vi "Dashboard Main.vi"() -> ()   [LabVIEW 2014]
uses:
  <vilib>/event_ctls.llb/eventvkey.ctl
  <vilib>/Rock Robotics/WPI/Dashboard/WPI_DashboardLogging Global.vi
  <vilib>/Rock Robotics/Network Tables/SD Read Numeric Array.vi
  <vilib>/Rock Robotics/Network Tables/SD Write Numeric Array.vi
  <vilib>/Rock Robotics/Network Tables/SD Write String Array.vi
  <vilib>/Rock Robotics/Network Tables/SD Read String Array.vi
  <vilib>/Rock Robotics/Network Tables/SD Write Boolean.vi
  <vilib>/Utility/config.llb/Write Key (String).vi
  <vilib>/Utility/config.llb/Write Key (I32).vi
  <vilib>/Utility/config.llb/NI_LVConfig.lvlib
panel:
  in  "TCP":refnum<k5>
  out "Camera IP":string
  out "Image Message":string="Timeout in Camera Communications"
  in  "Dashboard Tab":T1(tab)
  out "LR":dbl(slide) scale=-1.0..1.0
  out "RR":dbl(slide) scale=-1.0..1.0
  out "RF":dbl(slide) scale=-1.0..1.0
  out "LF":dbl(slide) scale=-1.0..1.0
  in  "Camera Settings":T2={"Frame Rate"=30, "Compression"=30, "Size"=1} {"Frame Rate" scale=1.0..30.0; "Size" items=["640x480", "320x240", "160x120"]}
  out "Mode":T3(ring)=enum."Auto Disabled"
  in  "DB Camera Config":bool
  out "fps":dbl format="%#.1g"
  out "Mbps":dbl format="%#.1g"
  out "Mbps 2":bool
  out "HID":T4(array[cluster])
  out "Time until start/end":sgl
  in  "DB/String 9":string
  in  "DB/String 8":string
  in  "DB/String 7":string
  in  "DB/String 6":string
  in  "DB/String 5":string
  in  "DB/String 4":string
  in  "DB/String 3":string
  in  "DB/String 2":string
  in  "DB/String 1":string
  in  "DB/String 0":string
  in  "DB/Slider 0":dbl(slide) scale=0.0..5.0
  in  "DB/Slider 1":dbl(slide) scale=0.0..5.0
  in  "DB/Slider 2":dbl(slide) scale=0.0..5.0
  in  "DB/Slider 3":dbl(slide) scale=0.0..5.0
  out "DB/LED 3":bool
  out "DB/LED 2":bool
  out "DB/LED 1":bool
  out "DB/LED 0":bool
  in  "DB/Button 3":bool
  in  "DB/Button 2":bool
  in  "DB/Button 1":bool
  in  "DB/Button 0":bool caption="New Name"
  in  "Rec Mode":enum32{"Stop", "Record", "Playback"}(radio)
  in  "Vision":u16(ring) items=["Camera Off", "USB Camera SW", "USB Camera HW", "IP Camera"]
  in  "Translate X":T5(ring)
  in  "Translate Y":T5(ring)=enum."Y left"
  in  "Rotate":T5(ring)=enum."X right"
  in  "Gyro Reset":T6(ring)
  in  "Toggle Field Centric":T6(ring)=enum."Trigger Right"
  in  "Low elevator":T7(ring)=enum."Left bumper"
  in  "Axis for manual Control of \narm":T8(ring)
  in  "High elevator":T7(ring)=enum."Right bumper"
  in  "Claw up":T7(ring)
  in  "Claw Down":T7(ring)=enum."B"
  in  "Axis for manual Control of Claw":T8(ring)
  in  "Rotate Claw":T9(ring)=enum."Right trigger"
  in  "Open/Close claw":T7(ring)=enum."Y"
  in  "Test Slider":dbl(slide) scale=0.0..100.0 scale format="%#_3g"
  in  "On/Off":bool caption="Solenoid"
  in  "Test Name":u16(ring) items=["Select the test to run...", "Example Test", "-------------------------------", "List of tests is built in robot code.", "Replace with your own automated tests."]
  in  "Test Tree":string(tree)
  in  "Motor":cluster{"Value":dbl, "Enable":bool} {"Value" scale=-1.0..1.0 scale format="%#_3g"}
  out "Progress":T10 {"Test Progress" scale=0.0..100.0}
  in  "Rev/Fwd":cluster{"Forward":bool, "Reverse":bool}
  in  "Test Ring":u16(ring) items=["Monochrome", "Color"]
  in  "Listbox":i32(listbox)
  in  "?":bool
  in  "Variables":string[](array[string])
  out "Camera Image":T11(plugin-control)
  out "Boolean":bool
  # "Battery"
  # "Primary Driver"
  # "Axis controls"
  # "Button Controls"
  # "Secondary Driver"
  # "Axis controls"
  # "Button Controls"
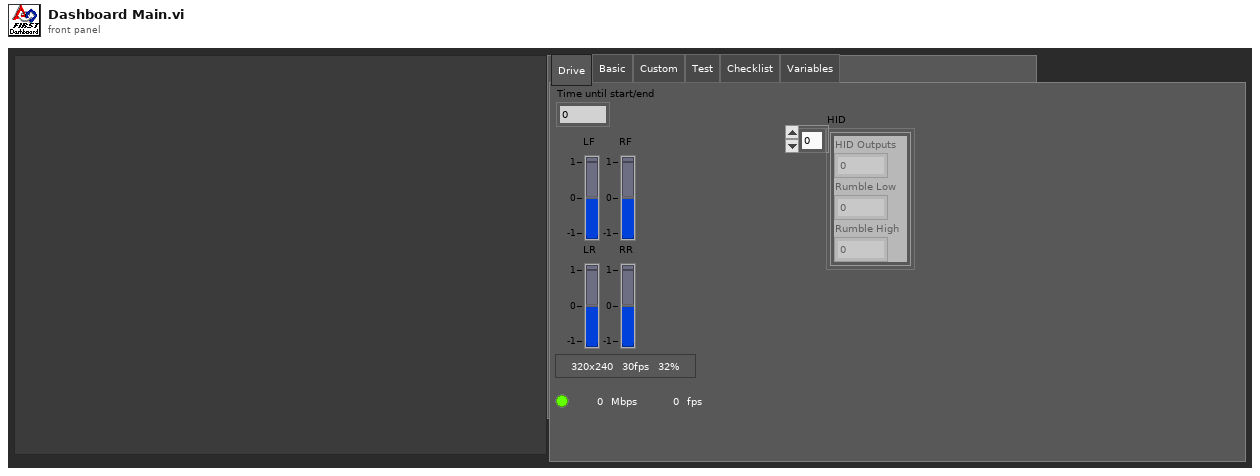
[diagram p1: front panel]
types:
  T1 = enum32{"Drive", "Basic", "Custom", "Test", "Checklist", "Variables"}
  T2 = cluster{"Frame Rate":i32, "Compression":i32, "Size":u16}
  T3 = enum8{"Tele-Op Disabled", "Tele-Op Enabled", "Auto Disabled", "Auto Enabled", "Test Disabled", "Test Enabled", "Disconnected", "No Code", "E-Stop"}
  T4 = cluster{"HID Outputs":u32, "Rumble Low":u16, "Rumble High":u16}[]
  T5 = enum16{"X left ", "Y left", "Z left", "X right", "Y right", "Z right"}
  T6 = enum16{"Trigger Left", "2 Left", "3 Left", "4 Left", "5 Left", "6 Left", "7 Left", "8 Left", "9 Left", "10 Left", "11 Left", "Trigger Right", "2 Right", "3 Right", "4 Right", "5 Right", "6 Right", "7 Right", "8 Right", "9 Right", "10 Right", "11 Right"}
  T7 = enum16{"A", "B", "X", "Y", "Left bumper", "Right bumper", "Back", "Start", "Left Joystick down", "Right Joystick down"}
  T8 = enum16{"Left X", "Left Y", "Left trigger", "R trigger", "R X", "R Y"}
  T9 = enum16{"Left X", "Left Y", "Left trigger", "Right trigger", "Right X", "Right Y"}
  T10 = cluster{"Test Progress":u8, "Test Progress Text":string}
  T11 = typedef "IMAQ Image.ctl" = refnum<image>
  T12 = typedef "Image Type" = u32
  T13 = cluster{"Error Strings":string, "Disable Counts":cluster{u16, u16}, "Rail Faults":cluster{u16, u16, u16}, "Robot IP":string, "DB Mode":u8, "Event Info":cluster{"Name":string, "Type":u8, "Number":u16, "Replay":u8}, "Camera Addr":string}
  T14 = cluster{"Storage":cluster{"Disk Free":u64, "RAM Block":u32, "RAM free":u32}, "CPU Utilization":cluster{"CPU % ISR":sgl, "CPU % Time Crit":sgl, "CPU % Timed Str":sgl, "CPU % High":sgl, "CPU % Above":sgl, "CPU % Normal":sgl, "CPU % Low":sgl}, "CAN":cluster{"% Bus Utilization":sgl, "Bus Off Cnt":u32, "TX_FIFO Full Cnt":u32, "Receive Error Cnt":u8, "Transmit Error Cnt":u8}, "HID":cluster{"HID Outputs":u32, "Rumble Low":u16, "Rumble High":u16}[]}
  T15 = cluster{"Status bits":cluster{"Test Mode":bool, "Autonomous":bool, "Enabled":bool, "Code Start":bool, "Brownout":bool, "Reserved 2":bool, "Reserved 3":bool, "E-Stop":bool}, "Code Trace":cluster{"Disabled":bool, "TeleOp":bool, "Auto":bool, "Test":bool}, "Controller Type":enum16{"unknown", "cRIO", "roboRio"}, "Code?":enum16{"unknown", "noCode", "code"}, "Battery V":dbl}
  T16 = cluster{"Control Bits":cluster{"TestMode":bool, "Autonomous":bool, "Enabled":bool, "FMS Present":bool, bool, bool, bool, "E-Stop":bool}, "Team Station ":u8, "Countdown":sgl, "Joystick Values":cluster{"Axes":dbl[], "Buttons":bool[], "POVs":i16[]}[]}
  T17 = enum16{"X left ", "Y left", "Z left", "X right", "Y right", "Z right"}[]
  T18 = enum16{"A", "B", "X", "Y", "Left bumper", "Right bumper", "Back", "Start", "Left Joystick down", "Right Joystick down"}[]
  T19 = enum16{"Trigger Left", "2 Left", "3 Left", "4 Left", "5 Left", "6 Left", "7 Left", "8 Left", "9 Left", "10 Left", "11 Left", "Trigger Right", "2 Right", "3 Right", "4 Right", "5 Right", "6 Right", "7 Right", "8 Right", "9 Right", "10 Right", "11 Right"}[]
  T20 = typedef "NI_LVConfig.lvlib/Config Data RefNum.ctl" = refnum<k1>
  T21 = cluster{"Operation":enum16{"Update", "Clear"}, "Color Box":u32}[]
  T22 = typedef "eventvkey.ctl" = enum16{"ASCII", "Enter", "Return", "Shift", "Ctrl", "Alt", "Cmd", "Opt", "Caps", "NumLock", "Clear", "Break", "Up", "Down", "Left", "Right", "Insert", "Delete", "Home", "End", "PageUp", "PageDown", "Escape", "Help", "Pause", "ScrollLock", "F1", "F2", "F3", "F4", "F5", "F6", "F7", "F8", "F9", "F10", "F11", "F12", "F13", "F14", "F15", "F16", "F17", "F18", "F19", "F20", "F21", "F22", "F23", "F24", "Play", "VolumeUp", "VolumeDown", "Mute", "Two Byte Char"}
  T23 = cluster{"Image Size":bool, "Image Type":bool, "Pixel Value":bool, "ROI Information":bool, "Zoom Factor":bool}
  T24 = enum8{"Enabled", "Disabled", "Disabled and Grayed Out"}
  T25 = cluster{"Operation":enum16{"Update", "Clear"}, "Color Box":u32}
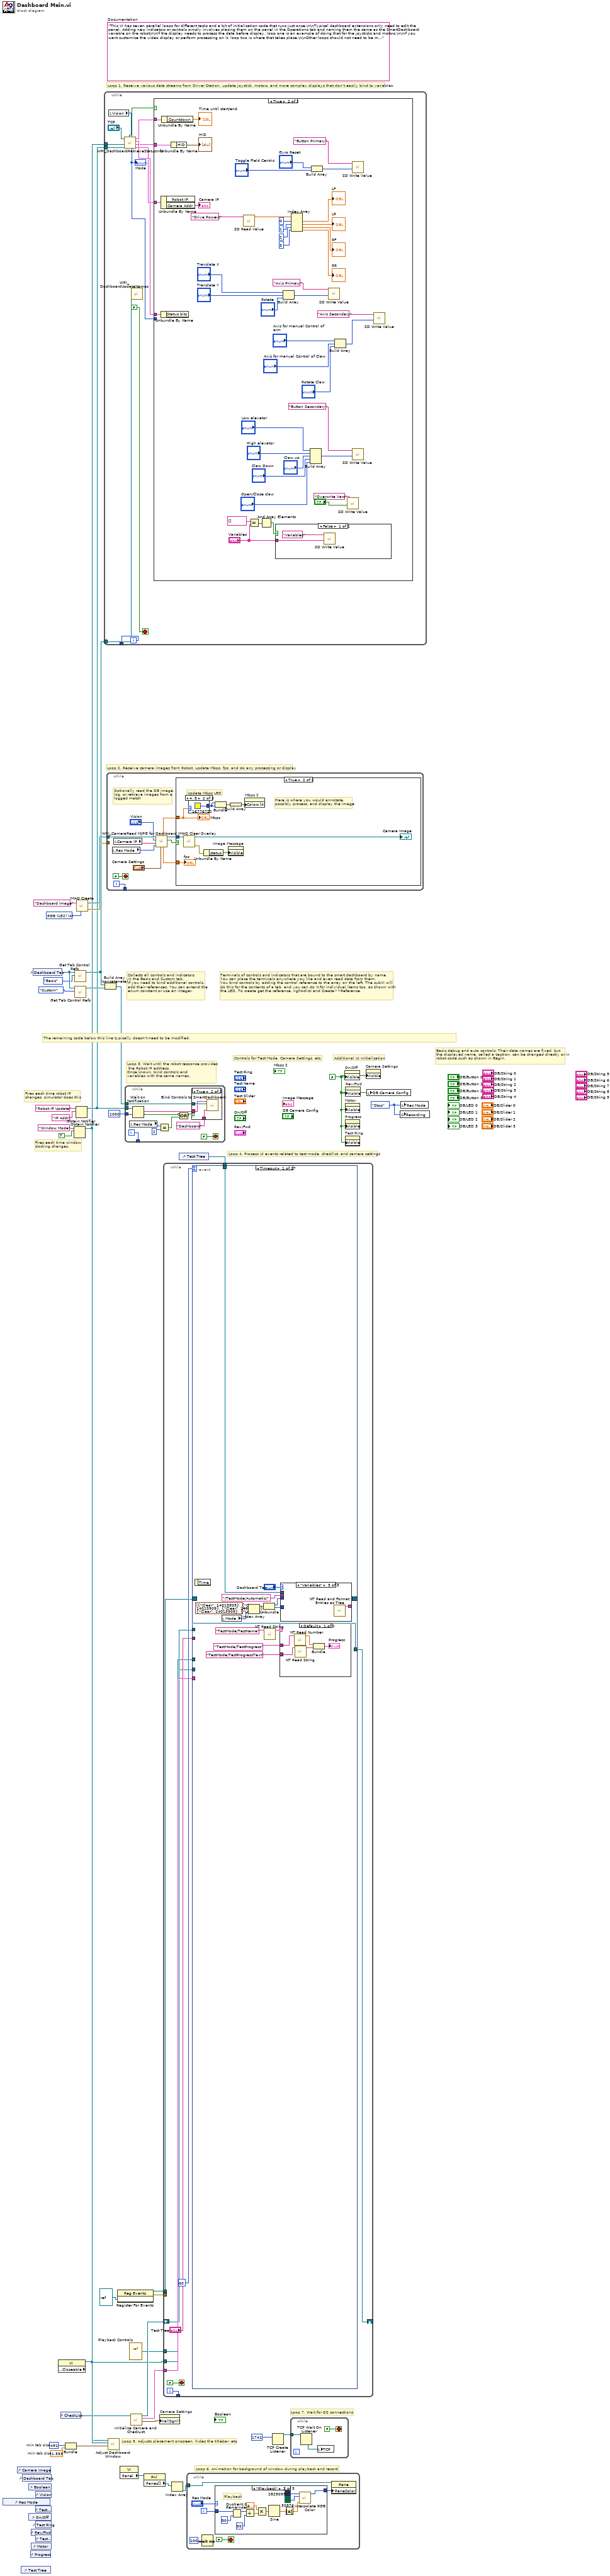
[diagram p0: block diagram]
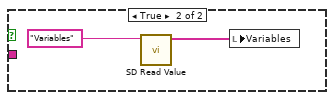
[diagram p3: hidden frame]
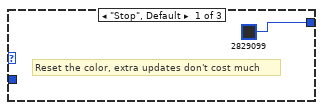
[diagram p4: hidden frame]
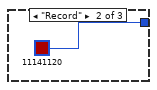
[diagram p5: hidden frame]
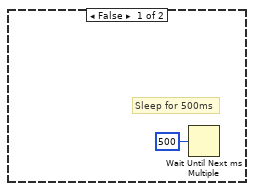
[diagram p7: hidden frame]
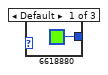
[diagram p8: hidden frame]
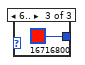
[diagram p9: hidden frame]
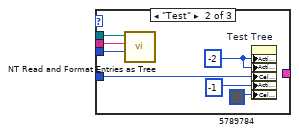
[diagram p11: hidden frame]
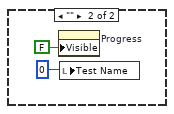
[diagram p12: hidden frame]
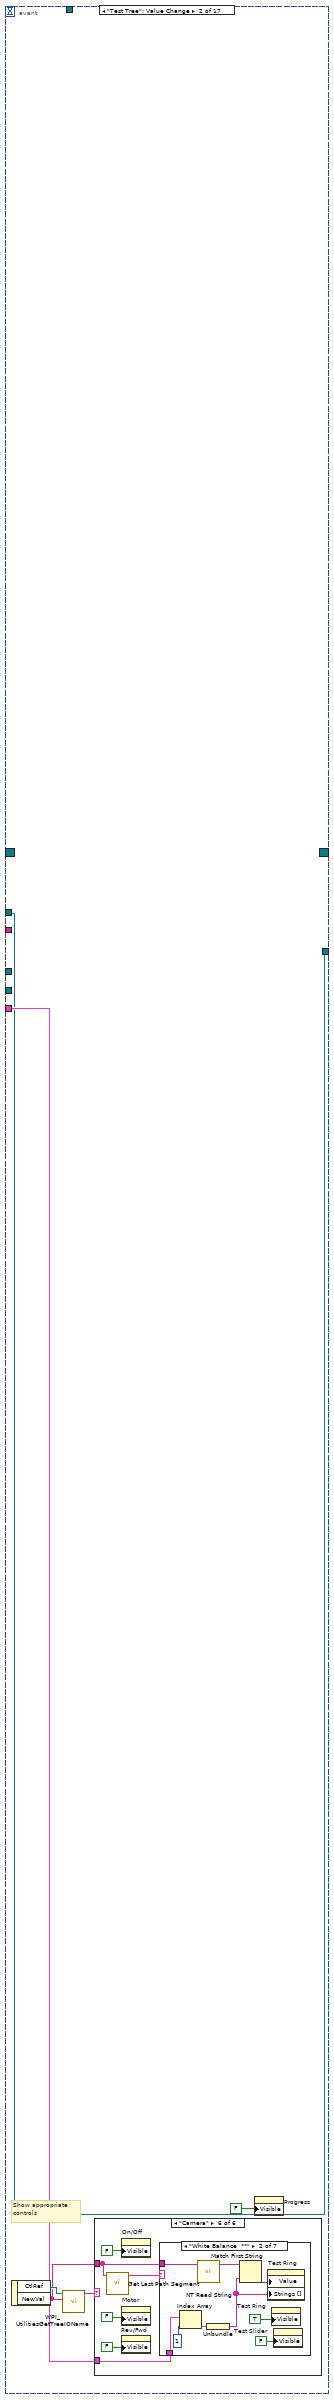
[diagram p13: hidden frame]
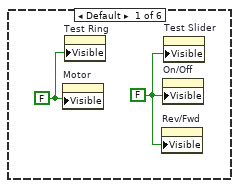
[diagram p14: hidden frame]
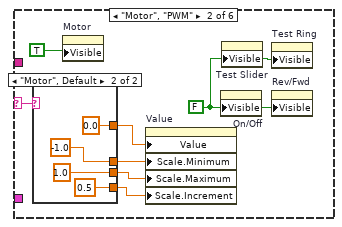
[diagram p15: hidden frame]
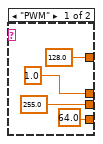
[diagram p16: hidden frame]
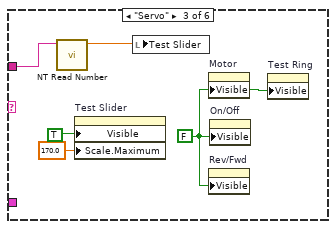
[diagram p17: hidden frame]
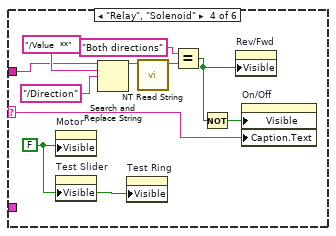
[diagram p18: hidden frame]
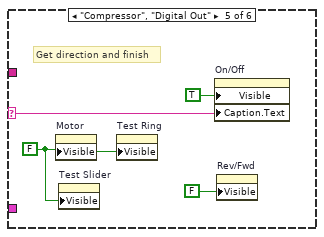
[diagram p19: hidden frame]
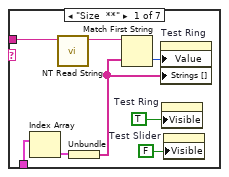
[diagram p20: hidden frame]
diagram:
  w12 = 491  # min tab size
  w11 = 1.333  # min tab size
  w17 = enum32{"Stop", "Record", "Playback"}."Stop" ("Rec Mode")
  w6 = FALSE ("Visible")
  (unwired) "This VI has seven parallel loops for different tasks and a bit of initialization code that runs just once.\n\nTypical dashboard extensions only need to edit the panel. Adding new indicators or controls simply involves placing them on the panel in the Operations tab and naming them the same as the SmartDashboard variable on the robot\n\nIf the display needs to process the data before display, loop one is an example of doing that for the joysticks and motors.\n\nIf you want customize the video display or perform processing on it, loop two is where that takes place.\n\nOther loops should not need to be modified. They are pretty standard, and document the task they perform."  # Documentation
  w37 = T12 4 items=["Grayscale (U8)", "Grayscale (I16)", "Grayscale (SGL)", "Complex (CSG)", "RGB (U32)", "HSL (U32)", "RGB (U64)"] ("Image Type")
  # "Loop 7. Wait for DS connections"
  # "Basic debug and auto controls: Their data names are fixed, but\nthe displayed name, called a caption, can be changed directly or in\nrobot code such as shown in Begin."
  # "Controls for Test Mode, Camera Settings, etc."
  # "Additional UI Initialization"
  # "Loop 6. Animation for background of window during playback and record"
  # "Fires each time robot IP\nchanges, simulator does this"
  # "Fires each time window\ndocking changes."
  # "Collects all controls and indicators\nin the Basic and Custom tab.\nIf you need to bind additional controls,\nadd their references. You can extend the\nenum constant or use an integer."
  # "The remaining code below this line typically doesn't need to be modified."
  # "Loop 4. Process UI events related to test mode, checklist, and camera settings"
  # "Terminals of controls and indicators that are bound to the smart dashboard by name.\nYou can place the terminals anywhere you like and even read data from them.\nYou bind controls by adding the control reference to the array on the left. The subVI will\ndo this for the contents of a tab, and you can do it for individual items too, as shown with\nthe LED. To create get the reference, right-click and Create>>Reference."
  # "Loop 3. Wait until the robot response provides\n the Robot IP address.\nOnce known, bind controls and\nvariables with the same names."
  # "Loop 5. Adjusts placement onscreen, hides the titlebar, etc."
  # "Loop 1. Receive various data streams from Driver Station, update joystick, motors, and more complex displays that don't easily bind to variables."
  # "Loop 2. Receive camera images from Robot, update Mbps, fps, and do any processing or display"
  n1 = control-ref of="Rec Mode"() -> ()  [unwired: 1 out]
  n2 = control-ref of="Camera Image"() -> ()  [unwired: 1 out]
  n3 = control-ref of="Test Tree"() -> ()  [unwired: 1 out]
  n4 = control-ref of="Dashboard Tab"() -> ()  [unwired: 1 out]
  n5 = control-ref of="Boolean"() -> ()  [unwired: 1 out]
  n6 = control-ref of="On/Off"() -> ()  [unwired: 1 out]
  n7 = control-ref of="Progress"() -> ()  [unwired: 1 out]
  n8 = control-ref of="Rev/Fwd"() -> ()  [unwired: 1 out]
  n9 = control-ref of="Motor"() -> ()  [unwired: 1 out]
  n10 = control-ref of="Dashboard Tab"() -> (w15:refnum<vi>)
  n11 = control-ref of="Test Slider"() -> ()  [unwired: 1 out]
  n12 = control-ref of="Vision"() -> ()  [unwired: 1 out]
  n13 = control-ref of="Test Ring"() -> ()  [unwired: 1 out]
  n14 = control-ref of="Test Name"() -> ()  [unwired: 1 out]
  n15 = property class="VI" props=["Front Panel.Closeable"]() -> (reference out=w16:refnum<vi>)  [unwired: 2 in, 2 out]
  n16 = control-ref of="CheckList"() -> (w7:refnum<vi>)
  n17 = Bundle("min tab size"=w12, "min tab size"=w11) -> (w10:cluster{"min tab size":i32, "min tab size":dbl})  [unwired: 1 in]
  n18 = Obtain Notifier(name (unnamed)="Window Mode", notification data type=TRUE) -> (notifier out=w3:refnum<notifier>)  [unwired: 2 in, 2 out]
  n19 = call <vilib>:"Get Tab Control Refs.vi"("Page Index"=T1."Basic" ("Dashboard Tab"), "TabControl in"=w15) -> ("ControlsOnPage"=w4:refnum<vi>[])  [unwired: 9 in]
  n20 = call <vilib>:"Get Tab Control Refs.vi"("Page Index"=T1."Custom" ("Dashboard Tab"), "TabControl in"=w15) -> ("ControlsOnPage"=w14:refnum<vi>[])  [unwired: 9 in]
  n21 = Obtain Notifier(name (unnamed)="Robot IP Update", notification data type="IP Addr" ("name (unnamed)")) -> (notifier out=w5:refnum<notifier>)  [unwired: 2 in, 2 out]
  n22 = call "IMAQ Create"("Image Name"="Dashboard Image", "Image Type"=w37) -> ("New Image"=w35:T11, "error out"=w34:errorcluster)  [unwired: 2 in, 1 out]
  n23 = while {
    tunnel: [w49] -> _
    tunnel: w5 -> [w43]
    tunnel: w4 -> [w42]
    tunnel: w3 -> [w38]
    i -> [w49]
    stop <- FALSE stop-if-true
    n24 = local read "Vision"() -> (w40:u16)
    n25 = call <vilib>:"WPI_DashboardRetrieveStatusInfo.vi"("Vision"=w40, "Binding Refnum"=w43, "Window Mode Notifier"=w38, "TCP Cnx"="TCP") -> ("Power and Errors"=w44:T13, "Robot Metrics"=w47:T14, "Status Info"=w48:T15, "Control Info"=w45:T16, "Robot Mode"=w41:T3, "Process?"=w46:bool)  [unwired: 2 in]
    "Mode" <- w41
    n26 = call <vilib>:"WPI_DashboardUpdateNames.vi"("Controls on Tab"=w42) -> ()  [unwired: 11 in]
    n27 = case shown="True" w46 {
      tunnel: w48 -> [_ w94]
      tunnel: w47 -> [_ w93]
      tunnel: w45 -> [_ w92]
      tunnel: w44 -> [_ w91]
      tunnel: w41 -> [_ _]
      frame False {
      }
      frame True {
        n28 = Unbundle By Name(w91) -> ("Camera Addr"=→"Camera IP":string)  [unwired: 1 out]
        n29 = Unbundle By Name(w94) -> ()  [unwired: 1 out]
        n30 = Unbundle By Name(w92) -> ("Countdown"=→"Time until start/end":sgl)
        n31 = Unbundle By Name(w93) -> ("HID"=→"HID":T4)
        n32 = call-poly <vilib>:"SD Read Value.vi"("Name"="Drive Powers") -> ("Numeric Array"=w86:dbl[])  [unwired: 8 in, 2 out]
        n33 = Equal?(x=string[] [], y="Variables") -> (x = y?=w55:bool[])
        n34 = And Array Elements(Boolean array=w55) -> (logical AND=w54:bool)
        n35 = case shown="False" w54 {
          tunnel: "Variables" -> [w95 _]
          frame False {
            n36 = call-poly <vilib>:"SD Write Value.vi"("String Array"=w95, "Name"="Variables") -> ()  [unwired: 8 in, 2 out]
          }
          frame True {
            n37 = call-poly <vilib>:"SD Read Value.vi"("Name"="Variables") -> ("String Array"=w97:string[])  [unwired: 9 in, 1 out]
            n38 = local write "Variables"(w97) -> ()
          }
        }
        n39 = Build Array("Translate X", "Translate Y", "Rotate") -> (w75:T17)
        n40 = Index Array(array=w86, index #1=0 ("index"), index #2=1 ("index"), index #3=2 ("index"), index #4=3 ("index")) -> (element #1=→"LF":dbl, element #2=→"LR":dbl, element #3=→"RF":dbl, element #4=→"RR":dbl)
        n41 = Build Array("Low elevator", "High elevator", "Claw up", "Claw Down", "Open/Close claw") -> (w66:T18)
        n42 = Build Array("Gyro Reset", "Toggle Field Centric") -> (w71:T19)
        n43 = call-poly <vilib>:"SD Write Value.vi"("Numeric Array"=w75, "Name"="Axis Primary") -> ()  [unwired: 8 in, 2 out]
        n44 = Build Array("Axis for manual Control of \narm", "Axis for manual Control of Claw", "Rotate Claw") -> (w68:u16[])
        n45 = call-poly <vilib>:"SD Write Value.vi"("Boolean"="?", "Name"="Overwrite Vars") -> ()  [unwired: 8 in, 2 out]
        n46 = call-poly <vilib>:"SD Write Value.vi"("Numeric Array"=w71, "Name"="Button Primary") -> ()  [unwired: 8 in, 2 out]
        n47 = call-poly <vilib>:"SD Write Value.vi"("Numeric Array"=w66, "Name"="Button Secondary") -> ()  [unwired: 8 in, 2 out]
        n48 = call-poly <vilib>:"SD Write Value.vi"("Numeric Array"=w68, "Name"="Axis Secondary") -> ()  [unwired: 8 in, 2 out]
      }
    }
  }
  n49 = Build Array (concatenate)(w4, w14) -> (w13:refnum<vi>[])
  n50 = while {
    tunnel: w35 -> [w107]
    tunnel: w34 -> [_]
    tunnel: [w108] -> _
    i -> [w108]
    stop <- FALSE stop-if-true
    # "Optionally read the DB image,\nlog, or retrieve images from a\nlogged match"
    n51 = local read "Rec Mode"() -> (w101:enum32{"Stop", "Record", "Playback"})
    n52 = local read "Camera IP"() -> (w99:string)
    n53 = call <vilib>:"WPI_CameraRead MJPG for Dashboard.vi"("Camera Settings"="Camera Settings", "Rec Mode"=w101, "Camera IP"=w99, "Camera Mode"="Vision", "Refnum in"=w107) -> ("Active"=w105:bool, "Refnum out"=w106:T11, "FPS"=w104:dbl, "Bandwidth (Mbps)"=w103:dbl)  [unwired: 3 in]
    n54 = case shown="True" w105 {
      tunnel: w106 -> [_ w114]
      tunnel: w103 -> [_ w113]
      tunnel: w104 -> [_ w111]
      frame False {
        # "Sleep for 500ms"
        n55 = Wait Until Next ms Multiple(millisecond multiple=u32 500) -> ()  [unwired: 1 out]
      }
      frame True {
        # "Here is where you would annotate,\npossibly process, and display the image"
        # "Update Mbps LED"
        n56 = call "IMAQ Clear Overlay"("Image"=w114) -> ("error out"=w118:errorcluster, "Image Out"=→"Camera Image":T11)  [unwired: 2 in, 7 out]
        n57 = case shown="4, 5" w113 {
          tunnel: [u32 6618880 ("Color Box") u32 16776722 ("Color Box") u32 16716800 ("Color Box")] -> w115
          frame Default {
          }
          frame 4, 5 {
          }
          frame 6.. {
          }
        }
        n58 = Unbundle By Name(w118) -> ("status"=w119:bool)
        n59 = Bundle("Color Box"=w115, "Color Box"=w115) -> (w117:cluster{"Color Box":u32, "Color Box":u32})  [unwired: 1 out]
        n60 = property on="Image Message" class="Str"("Visible"=w119) -> ()  [unwired: 2 in, 2 out]
        n61 = Build Array(w117) -> (w116:cluster{"Color Box":u32, "Color Box":u32}[])
        n62 = property on="Mbps 2" class="Bool (strict)"("Colors [4]"=w116) -> ()  [unwired: 2 in, 2 out]
        "Mbps" <- w113
        "fps" <- w111
      }
    }
  }
  n63 = call "Adjust Dashboard Window.vi"("Size Constraints"=w10, "VI"=w16, "Notifier in"=w3) -> ()  [unwired: 9 in]
  n64 = register-events(refnum<vi> refnum) -> (reference out=w21:refnum<event-registration>, error out=w20:errorcluster)  [unwired: 2 in]
  n65 = property class="VI"() -> ("Panel"=w24:refnum<vi>)  [unwired: 2 in, 2 out]
  n66 = while {
    tunnel: w13 -> [w134]
    tunnel: w5 -> [w132]
    tunnel: [w130] -> _
    tunnel: u32 1000 ("milliseconds to wait") -> [w129]
    i -> [w130]
    stop <- FALSE stop-if-true
    n67 = local read "Rec Mode"() -> (w125:enum32{"Stop", "Record", "Playback"})
    n68 = Wait on Notification(notifier=w132, timeout in ms (-1)=w129) -> (notification=w131:string, timed out?=w127:bool)  [unwired: 2 in, 2 out]
    n69 = Equal?(x=w125, y=u16 2 ("Rec Mode")) -> (x = y?=w126:bool)
    n70 = Compound Arithmetic op=OR(invert w127, w126) -> (w128:bool)
    n71 = case shown="True" w128 {
      tunnel: w134 -> [_ w137]
      tunnel: w131 -> [_ w136]
      tunnel: "Dashboard" -> [_ w135]
      frame False {
      }
      frame True {
        n72 = call <vilib>:"Bind Controls to SmartDashboard.vi"("Client Name"=w135, "Bound Control Refs"=w137, "Server IP Address"=w136) -> ()  [unwired: 9 in]
      }
    }
  }
  n73 = vi-ref "Playback Controls.vi"() -> (w22:refnum<vi>)
  n74 = call "Initialize Camera and CheckList.vi"("ListBox in"=w7) -> ("Cluster"=w28:cluster{"value":i32, "value":i32, "index":i32}, "Array"=w29:cluster{string[]}[], "File Refnum"=w27:T20)  [unwired: 8 in]
  n75 = property class="Pnl"(reference=w24) -> ("Panes[]"=w25:refnum<vi>[])  [unwired: 1 in, 2 out]
  n76 = property on="Camera Settings" class="Clust (strict)"("Val(Sgnl)"=w28) -> ()  [unwired: 2 in, 2 out]
  n77 = Index Array(array=w25) -> (element=w23:refnum<vi>)  [unwired: 1 in]
  n78 = control-ref of="Test Tree"() -> (w26:refnum<vi>)
  n79 = while {
    tunnel: w29 -> [w145]
    shift-right: [w144] -> _
    shift-left: w27 -> [w143]
    tunnel: [w142] -> _
    tunnel: w26 -> [w141]
    tunnel: w22 -> [w140]
    tunnel: w21 -> [w139]
    tunnel: w20 -> [_]
    tunnel: w16 -> [w138]
    i -> [w142]
    stop <- FALSE stop-if-true
    n80 = event shown="[0] Timeout" {
      selector: w139 -> [_ _ _ _ _ _ _ _ _ _ _ _ _ _ _ _ _]
      dyn-events: [_ _ _ _ _ _ _ _ _ _ _ _ _ w382 _ _ _] -> _
      timeout: u32 60 ("milliseconds to wait") -> [_ _ _ _ _ _ _ _ _ _ _ _ _ _ _ _ _]
      tunnel: w141 -> [w157 _ _ _ _ _ _ _ _ _ _ _ _ _ _ _ _]
      tunnel: "Test Tree" -> [_ _ _ _ _ _ _ _ w351 w359 w361 w365 w373 _ _ _ _]
      tunnel: w145 -> [_ w178 _ _ _ _ w315 w345 _ _ _ _ _ _ _ _ _]
      tunnel: [w153 w177 w276 w281 w289 w301 w314 w338 w350 w357 w360 w364 w372 w384 w398 w399 w409] -> w144
      tunnel: w143 -> [w153 w177 w276 w281 w289 w301 w313 w338 w350 w357 w360 w364 w372 w384 w398 w399 w409]
      tunnel: w140 -> [_ _ _ _ _ _ _ _ _ _ _ _ _ w385 _ w402 _]
      tunnel: w138 -> [_ _ _ _ _ _ _ _ _ _ _ _ _ w380 _ _ _]
      event Timeout {
        n81 = event-data() -> ()  [unwired: 1 in, 1 out]
        n82 = local read "Mode"() -> (w156:T3)
        n83 = Index Array(array=T21 [{"Operation"=enum."Clear", "Color Box"=14013909}, {"Operation"=enum."Clear", "Color Box"=14013909}, {"Operation"=enum."Clear", "Color Box"=14013909}, {"Operation"=enum."Clear", "Color Box"=14013909}, {"Operation"=enum."Update", "Color Box"=14013909}, {"Operation"=enum."Update", "Color Box"=16777215}, {"Operation"=enum."Clear", "Color Box"=14013909}, {"Operation"=enum."Clear", "Color Box"=14013909}, {"Operation"=enum."Clear", "Color Box"=14013909}], index=w156) -> (element=w151:T25)
        n84 = Unbundle(w151) -> ("Operation"=w150:enum16{"Update", "Clear"}, "Color Box"=w149:u32)
        n85 = call <vilib>:"NT Read String.vi"("Name"="TestMode/TestName") -> ("String"=w160:string)  [unwired: 9 in, 1 out]
        n86 = case shown="Default" w160 {
          tunnel: "TestMode/TestProgress" ("Name") -> [w171 _]
          tunnel: "TestMode/TestProgressText" ("Name") -> [w170 _]
          frame Default {
            n87 = call <vilib>:"NT Read Number.vi"("Name"=w171) -> ("Numeric"=w172:dbl)  [unwired: 9 in, 1 out]
            n88 = call <vilib>:"NT Read String.vi"("Name"=w170) -> ("String"=w173:string)  [unwired: 9 in, 1 out]
            n89 = Bundle("Numeric"=w172, "String"=w173) -> (→"Progress":cluster{"Numeric":dbl, "String":string})  [unwired: 1 in]
          }
          frame "" {
            n90 = property on="Progress" class="Clust (strict)"("Visible"=FALSE) -> ()  [unwired: 2 in, 2 out]
            n91 = local write "Test Name"(u16 0) -> ()
          }
        }
        n92 = case shown="\"Variables\"" "Dashboard Tab" {
          tunnel: w157 -> [_ w168 _]
          tunnel: "/TestMode/Automatic/" ("Name Pattern") -> [_ w167 _]
          tunnel: w150 -> [_ w166 _]
          tunnel: [_ _ w169] -> _
          tunnel: w149 -> [_ w162 _]
          frame "Custom", Default {
          }
          frame "Test" {
            w165 = -2 ("Active Item:Row Number")
            n93 = call <vilib>:"NT Read and Format Entries as Tree.vi"("Operation"=w166, "Name Pattern"=w167, "Tree Refnum"=w168) -> ()  [unwired: 7 in, 2 out]
            n94 = property on="Test Tree" class="Tree (strict)"("Active Item Row Number"=w165, "ActiveColNum"=w165, "CellBG"=w162, "Active Item Row Number"=-1 ("Active Item:Row Number"), "CellBG"=u32 5789784 ("Color Box")) -> ()  [unwired: 2 in, 2 out]
          }
          frame "Variables" {
            n95 = call <vilib>:"NT Read and Format Entries as Tree.vi"() -> ("Formatted Strings"=w169:cluster{"Name":string, "Value":string}[])  [unwired: 10 in, 1 out]
          }
        }
      }
      event "Test Tree": Value Change {
        # "Show appropriate\ncontrols"
        n96 = event-data() -> ("CtlRef"=w181:refnum<vi>, "NewVal"=w179:string)  [unwired: 1 in]
        n97 = call <vilib>:"WPI_UtilitiesGetTreeIOName.vi"("NewVal"=w179, "TreeControl in"=w181) -> ("I/O Name"=w182:string)  [unwired: 9 in]
        n98 = case shown="\"Camera\"" w182 {
          selector: w182 -> [_ w189 _ w207 w216 _]
          tunnel: w179 -> [_ _ w204 w206 _ w223]
          tunnel: w178 -> [_ _ _ _ _ w222]
          frame Default {
            w184 = FALSE ("Visible")
            w183 = FALSE ("Visible")
            n99 = property on="Motor" class="Clust (strict)"("Visible"=w183) -> ()  [unwired: 2 in, 2 out]
            n100 = property on="Test Ring" class="Ring (strict)"("Visible"=w183) -> ()  [unwired: 2 in, 2 out]
            n101 = property on="Rev/Fwd" class="Clust (strict)"("Visible"=w184) -> ()  [unwired: 2 in, 2 out]
            n102 = property on="On/Off" class="Bool (strict)"("Visible"=w184) -> ()  [unwired: 2 in, 2 out]
            n103 = property on="Test Slider" class="Slide (strict)"("Visible"=w184) -> ()  [unwired: 2 in, 2 out]
          }
          frame "Motor", "PWM" {
            w190 = FALSE ("Visible")
            n104 = case shown="\"Motor\", Default" w189 {
              tunnel: [1.0 ("Value") -1.0 ("Value")] -> w188
              tunnel: [255.0 ("Value") 1.0 ("Value")] -> w187
              tunnel: [128.0 ("Value") 0.0 ("Value")] -> w186
              tunnel: [64.0 ("Value") 0.5 ("Value")] -> w185
              frame "PWM" {
              }
              frame "Motor", Default {
              }
            }
            n105 = property on="Motor" class="Clust (strict)"("Visible"=TRUE) -> ()  [unwired: 2 in, 2 out]
            n106 = property on="Value" class="Slide (strict)"("Value"=w186, "Scale.Minimum"=w188, "Scale.Maximum"=w187, "Scale.Increment"=w185) -> ()  [unwired: 2 in, 2 out]
            n107 = property on="On/Off" class="Bool (strict)"("Visible"=w190) -> ()  [unwired: 2 in, 2 out]
            n108 = property on="Test Slider" class="Slide (strict)"("Visible"=w190) -> ()  [unwired: 2 in, 2 out]
            n109 = property on="Test Ring" class="Ring (strict)"("Visible"=w190) -> ()  [unwired: 2 in, 2 out]
            n110 = property on="Rev/Fwd" class="Clust (strict)"("Visible"=w190) -> ()  [unwired: 2 in, 2 out]
          }
          frame "Servo" {
            w202 = FALSE ("Visible")
            n111 = call <vilib>:"NT Read Number.vi"("Name"=w204) -> ("Numeric"=w203:dbl)  [unwired: 9 in, 1 out]
            n112 = property on="Test Slider" class="Slide (strict)"("Visible"=TRUE, "Scale.Maximum"=170.0 ("Scale.Range:Maximum")) -> ()  [unwired: 2 in, 2 out]
            n113 = local write "Test Slider"(w203) -> ()
            n114 = property on="Motor" class="Clust (strict)"("Visible"=w202) -> ()  [unwired: 2 in, 2 out]
            n115 = property on="Rev/Fwd" class="Clust (strict)"("Visible"=w202) -> ()  [unwired: 2 in, 2 out]
            n116 = property on="On/Off" class="Bool (strict)"("Visible"=w202) -> ()  [unwired: 2 in, 2 out]
            n117 = property on="Test Ring" class="Ring (strict)"("Visible"=w202) -> ()  [unwired: 2 in, 2 out]
          }
          frame "Relay", "Solenoid" {
            w205 = FALSE ("Visible")
            n118 = property on="Motor" class="Clust (strict)"("Visible"=w205) -> ()  [unwired: 2 in, 2 out]
            n119 = property on="Test Slider" class="Slide (strict)"("Visible"=w205) -> ()  [unwired: 2 in, 2 out]
            n120 = Search and Replace String(input string=w206, search string="/Value  **", replace string="/Direction") -> (result string=w212:string)  [unwired: 5 in, 3 out]
            n121 = property on="Test Ring" class="Ring (strict)"("Visible"=w205) -> ()  [unwired: 2 in, 2 out]
            n122 = call <vilib>:"NT Read String.vi"("Name"=w212) -> ("String"=w210:string)  [unwired: 9 in, 1 out]
            n123 = Equal?(x="Both directions", y=w210) -> (x = y?=w208:bool)
            n124 = Not(x=w208) -> (.not. x?=w209:bool)
            n125 = property on="Rev/Fwd" class="Clust (strict)"("Visible"=w208) -> ()  [unwired: 2 in, 2 out]
            n126 = property on="On/Off" class="Bool (strict)"("Visible"=w209, "Caption.Text"=w207) -> ()  [unwired: 2 in, 2 out]
          }
          frame "Compressor", "Digital Out" {
            w215 = FALSE ("Visible")
            # "Get direction and finish"
            n127 = property on="Motor" class="Clust (strict)"("Visible"=w215) -> ()  [unwired: 2 in, 2 out]
            n128 = property on="Test Slider" class="Slide (strict)"("Visible"=w215) -> ()  [unwired: 2 in, 2 out]
            n129 = property on="Test Ring" class="Ring (strict)"("Visible"=w215) -> ()  [unwired: 2 in, 2 out]
            n130 = property on="On/Off" class="Bool (strict)"("Visible"=TRUE, "Caption.Text"=w216) -> ()  [unwired: 2 in, 2 out]
            n131 = property on="Rev/Fwd" class="Clust (strict)"("Visible"=FALSE) -> ()  [unwired: 2 in, 2 out]
          }
          frame "Camera" {
            n132 = call <vilib>:"Get Last Path Segment.vi"("String in"=w223) -> ("String out"=w224:string)  [unwired: 10 in]
            n133 = property on="On/Off" class="Bool (strict)"("Visible"=FALSE) -> ()  [unwired: 2 in, 2 out]
            n134 = property on="Motor" class="Clust (strict)"("Visible"=FALSE) -> ()  [unwired: 2 in, 2 out]
            n135 = property on="Rev/Fwd" class="Clust (strict)"("Visible"=FALSE) -> ()  [unwired: 2 in, 2 out]
            n136 = case shown="\"White Balance  **\"" w224 {
              tunnel: w223 -> [w230 w239 w248 w257 w266 _ w272]
              tunnel: w222 -> [w228 w236 w245 w254 w263 _ _]
              frame "Size  **" {
                n137 = Index Array(array=w228) -> (element=w227:cluster{string[]})  [unwired: 1 in]
                n138 = call <vilib>:"NT Read String.vi"("Name"=w230) -> ("String"=w229:string)  [unwired: 9 in, 1 out]
                n139 = Unbundle(w227) -> (w225:string[])
                n140 = Match First String(2:w225, 3:w229) -> (0:w226:i32)  [unwired: 1 out]
                n141 = property on="Test Ring" class="Ring (strict)"("Value"=w226, "Strings []"=w225) -> ()  [unwired: 2 in, 2 out]
                n142 = property on="Test Ring" class="Ring (strict)"("Visible"=TRUE) -> ()  [unwired: 2 in, 2 out]
                n143 = property on="Test Slider" class="Slide (strict)"("Visible"=FALSE) -> ()  [unwired: 2 in, 2 out]
              }
              frame "White Balance  **" {
                n144 = Index Array(array=w236, index=1) -> (element=w237:cluster{string[]})
                n145 = call <vilib>:"NT Read String.vi"("Name"=w239) -> ("String"=w238:string)  [unwired: 9 in, 1 out]
                n146 = Unbundle(w237) -> (w234:string[])
                n147 = Match First String(2:w234, 3:w238) -> (0:w233:i32)  [unwired: 1 out]
                n148 = property on="Test Ring" class="Ring (strict)"("Value"=w233, "Strings []"=w234) -> ()  [unwired: 2 in, 2 out]
                n149 = property on="Test Ring" class="Ring (strict)"("Visible"=TRUE) -> ()  [unwired: 2 in, 2 out]
                n150 = property on="Test Slider" class="Slide (strict)"("Visible"=FALSE) -> ()  [unwired: 2 in, 2 out]
              }
              frame "Exposure  **" {
                n151 = Index Array(array=w245, index=2) -> (element=w246:cluster{string[]})
                n152 = call <vilib>:"NT Read String.vi"("Name"=w248) -> ("String"=w247:string)  [unwired: 9 in, 1 out]
                n153 = Unbundle(w246) -> (w242:string[])
                n154 = Match First String(2:w242, 3:w247) -> (0:w243:i32)  [unwired: 1 out]
                n155 = property on="Test Ring" class="Ring (strict)"("Value"=w243, "Strings []"=w242) -> ()  [unwired: 2 in, 2 out]
                n156 = property on="Test Ring" class="Ring (strict)"("Visible"=TRUE) -> ()  [unwired: 2 in, 2 out]
                n157 = property on="Test Slider" class="Slide (strict)"("Visible"=FALSE) -> ()  [unwired: 2 in, 2 out]
              }
              frame "Exposure Priority  **" {
                n158 = Index Array(array=w254, index=3) -> (element=w255:cluster{string[]})
                n159 = call <vilib>:"NT Read String.vi"("Name"=w257) -> ("String"=w256:string)  [unwired: 9 in, 1 out]
                n160 = Unbundle(w255) -> (w251:string[])
                n161 = Match First String(2:w251, 3:w256) -> (0:w252:i32)  [unwired: 1 out]
                n162 = property on="Test Ring" class="Ring (strict)"("Value"=w252, "Strings []"=w251) -> ()  [unwired: 2 in, 2 out]
                n163 = property on="Test Ring" class="Ring (strict)"("Visible"=TRUE) -> ()  [unwired: 2 in, 2 out]
                n164 = property on="Test Slider" class="Slide (strict)"("Visible"=FALSE) -> ()  [unwired: 2 in, 2 out]
              }
              frame "Color Enable  **" {
                n165 = Index Array(array=w263, index=4) -> (element=w264:cluster{string[]})
                n166 = call <vilib>:"NT Read String.vi"("Name"=w266) -> ("String"=w265:string)  [unwired: 9 in, 1 out]
                n167 = Unbundle(w264) -> (w260:string[])
                n168 = Match First String(2:w260, 3:w265) -> (0:w261:i32)  [unwired: 1 out]
                n169 = property on="Test Ring" class="Ring (strict)"("Value"=w261, "Strings []"=w260) -> ()  [unwired: 2 in, 2 out]
                n170 = property on="Test Ring" class="Ring (strict)"("Visible"=TRUE) -> ()  [unwired: 2 in, 2 out]
                n171 = property on="Test Slider" class="Slide (strict)"("Visible"=FALSE) -> ()  [unwired: 2 in, 2 out]
              }
              frame Default {
                n172 = property on="Test Ring" class="Ring (strict)"("Visible"=FALSE) -> ()  [unwired: 2 in, 2 out]
                n173 = property on="Test Slider" class="Slide (strict)"("Visible"=FALSE) -> ()  [unwired: 2 in, 2 out]
              }
              frame "Brightness  **", "Color Level  **", "Compression  **", "FPS  **", "Sharpness  **" {
                n174 = call <vilib>:"NT Read Number.vi"("Name"=w272) -> ("Numeric"=w271:dbl)  [unwired: 9 in, 1 out]
                n175 = local write "Test Slider"(w271) -> ()
                n176 = property on="Test Slider" class="Slide (strict)"("Visible"=TRUE, "Scale.Maximum"=100.0 ("Scale.Range:Maximum")) -> ()  [unwired: 2 in, 2 out]
                n177 = property on="Test Ring" class="Ring (strict)"("Visible"=FALSE) -> ()  [unwired: 2 in, 2 out]
              }
            }
          }
        }
        n178 = property on="Progress" class="Clust (strict)"("Visible"=FALSE) -> ()  [unwired: 2 in, 2 out]
      }
      event "Test Name": Mouse Enter {
        # "Populate the ring with the list of tests"
        n179 = event-data() -> ()  [unwired: 1 in, 1 out]
        n180 = call <vilib>:"NT Read String Array.vi"("Name"="TestMode/TestList") -> ("String Array"=w280:string[])  [unwired: 9 in, 1 out]
        n181 = Build Array (concatenate)("Select the test to run...", w280) -> (w279:string[])
        n182 = property on="Test Name" class="Ring (strict)"("Strings []"=w279) -> ()  [unwired: 2 in, 2 out]
      }
      event "Test Name": Value Change {
        w282 = FALSE ("Visible")
        # "Tell the robot the test name to run"
        n183 = event-data() -> ("NewVal"=w286:u16)  [unwired: 1 in]
        n184 = property on="Test Name" class="Ring (strict)"() -> ("Strings []"=w287:string[])  [unwired: 2 in, 2 out]
        n185 = local write "Progress"(T10 {"Test Progress"=0, "Test Progress Text"=""} ("Progress")) -> ()
        n186 = Index Array(array=w287, index=w286) -> (element=w285:string)
        n187 = call <vilib>:"NT Write String.vi"("String"=w285, "Name"="TestMode/TestName") -> ()  [unwired: 9 in, 1 out]
        n188 = property on="Progress" class="Clust (strict)"("Visible"=TRUE) -> ()  [unwired: 2 in, 2 out]
        n189 = property on="Motor" class="Clust (strict)"("Visible"=w282) -> ()  [unwired: 2 in, 2 out]
        n190 = property on="Test Slider" class="Slide (strict)"("Visible"=w282) -> ()  [unwired: 2 in, 2 out]
        n191 = property on="On/Off" class="Bool (strict)"("Visible"=w282) -> ()  [unwired: 2 in, 2 out]
        n192 = property on="Rev/Fwd" class="Clust (strict)"("Visible"=w282) -> ()  [unwired: 2 in, 2 out]
        n193 = property on="Test Ring" class="Ring (strict)"("Visible"=w282) -> ()  [unwired: 2 in, 2 out]
      }
      event "Listbox": Double Click {
        # "Shift clears all"
        # "Update symbols on the listbox"
        n194 = event-data() -> ("PlatMods.Shift"=w290:bool, "Row"=w292:i32)  [unwired: 1 in]
        n195 = case shown="True" w290 {
          tunnel: w292 -> [w296 _]
          tunnel: 1 -> [w295 _]
          frame False {
            n196 = property on="Listbox" class="LstBox (strict)"() -> ("Item Symbols"=w294:i32[])  [unwired: 2 in, 2 out]
            n197 = Replace Array Subset(array=w294, new element=w295, index=w296) -> (w293:i32[])
            n198 = property on="Listbox" class="LstBox (strict)"("Item Symbols"=w293) -> ()  [unwired: 2 in, 2 out]
          }
          frame True {
            w297 = 0 ("Top Row")
            n199 = property on="Listbox" class="LstBox (strict)"() -> ("Number of Rows"=w299:u32)  [unwired: 2 in, 2 out]
            n200 = Initialize Array(0, w299) -> (w298:i32[])
            n201 = property on="Listbox" class="LstBox (strict)"("Top Row"=w297, "Value"=w297, "Item Symbols"=w298) -> ()  [unwired: 2 in, 2 out]
          }
        }
      }
      event "Listbox": Key Down {
        # "Update symbols on the listbox\nLeft and right keys check and uncheck"
        n202 = event-data() -> ("VKey"=w303:T22)  [unwired: 1 in]
        n203 = case shown="\"Left\", \"Right\"" w303 {
          selector: w303 -> [w308 _]
          tunnel: eventvkey."Left" ("VKey") -> [w306 _]
          frame "Left", "Right" {
            n204 = Equal?(x=w306, y=w308) -> (x = y?=w307:bool)
            n205 = Select(t=0, s=w307, f=1) -> (s? t:f=w309:i32)
            n206 = property on="Listbox" class="LstBox (strict)"() -> ("Item Symbols"=w312:i32[])  [unwired: 2 in, 2 out]
            n207 = Replace Array Subset(array=w312, new element=w309, index="Listbox") -> (w311:i32[])
            n208 = property on="Listbox" class="LstBox (strict)"("Item Symbols"=w311) -> ()  [unwired: 2 in, 2 out]
          }
          frame Default {
          }
        }
      }
      event "DB Camera Config": Value Change {
        # "Show or hide the cluster of controls, store in ini file"
        n209 = event-data() -> ("NewVal"=w316:bool)  [unwired: 1 in]
        n210 = case shown="False" w316 {
          tunnel: w315 -> [w325 _]
          tunnel: [w318 w336] -> w314
          tunnel: w313 -> [w317 w336]
          frame False {
            w332 = "Camera"
            w335 = FALSE ("Visible")
            n211 = local read "Camera Settings"() -> (w324:T2)
            n212 = Index Array(array=w325) -> (element=w328:cluster{string[]})  [unwired: 1 in]
            n213 = Unbundle(w324) -> ("Frame Rate"=w323:i32, "Compression"=w322:i32, "Size"=w326:u16)
            n214 = Unbundle(w328) -> (w327:string[])
            n215 = Index Array(array=w327, index=w326) -> (element=w321:string)
            n216 = call-poly <vilib>:"Write Key.vi"("section"=w332, "value"=w321, "key"="Size", "refnum"=w317) -> ("refnum out"=w334:T20)  [unwired: 2 in, 5 out]
            n217 = call-poly <vilib>:"Write Key.vi"("section"=w332, "value"=w323, "key"="FrameRate", "refnum"=w334) -> ("refnum out"=w333:T20)  [unwired: 1 in, 6 out]
            n218 = property on="Camera Settings" class="Clust (strict)"("Visible"=w335) -> ()  [unwired: 2 in, 2 out]
            n219 = local write "DB Camera Config"(w335) -> ()
            n220 = call-poly <vilib>:"Write Key.vi"("section"=w332, "value"=w322, "key"="Compression", "refnum"=w333) -> ("refnum out"=w319:T20)  [unwired: 1 in, 6 out]
            n221 = call <vilib>:"Close Config Data.vi"("refnum"=w319) -> ("file path"=w320:path)  [unwired: 2 in, 8 out]
            n222 = call <vilib>:"Open Config Data.vi"("configuration file path"=w320) -> ("refnum"=w318:T20)  [unwired: 8 in, 2 out]
          }
          frame True {
            n223 = property on="Camera Settings" class="Clust (strict)"("Visible"=TRUE) -> ()  [unwired: 2 in, 2 out]
          }
        }
      }
      event "Camera Settings": Value Change {
        # "Update summary string when any elements of DB camera change"
        n224 = event-data() -> ("NewVal"=w349:T2)  [unwired: 1 in]
        n225 = Index Array(array=w345) -> (element=w344:cluster{string[]})  [unwired: 1 in]
        n226 = Unbundle(w349) -> ("Frame Rate"=w340:i32, "Compression"=w339:i32, "Size"=w342:u16)
        n227 = Unbundle(w344) -> (w343:string[])
        n228 = Index Array(array=w343, index=w342) -> (element=w341:string)
        n229 = Format Into String(format string="%s   %dfps   %d%%", w341, w340, w339) -> (resulting string=w346:string)  [unwired: 2 in, 1 out]
        n230 = Build Array(w346) -> (w347:string[])
        n231 = property on="DB Camera Config" class="Bool (strict)"("Strings [4]"=w347) -> ()  [unwired: 2 in, 2 out]
      }
      event "Motor.Enable": Value Change {
        # "When the test mode otor enable helper is set, update that\ntree row item's value"
        n232 = event-data() -> ("NewVal"=w355:bool)  [unwired: 1 in]
        n233 = Unbundle("Motor") -> ("Value"=w354:dbl)  [unwired: 1 out]
        n234 = Select(t=w354, s=w355, f=0.0) -> (s? t:f=w352:dbl)
        n235 = call <vilib>:"NT Write Number.vi"("Numeric"=w352, "Name"=w351) -> ()  [unwired: 9 in, 1 out]
      }
      event "Test Slider": Value Change {
        # "When the test mode slider helper is set, update that\ntree row item's value"
        n236 = event-data() -> ("NewVal"=w358:dbl)  [unwired: 1 in]
        n237 = call <vilib>:"NT Write Number.vi"("Numeric"=w358, "Name"=w359) -> ()  [unwired: 9 in, 1 out]
      }
      event "On/Off": Value Change {
        # "When the test mode on/off helper value is set, update that\ntree row item's value"
        n238 = event-data() -> ("NewVal"=w363:bool)  [unwired: 1 in]
        n239 = Boolean To (0,1)(Boolean=w363) -> (0, 1=w362:i16)
        n240 = call <vilib>:"NT Write Number.vi"("Numeric"=w362, "Name"=w361) -> ()  [unwired: 9 in, 1 out]
      }
      event "Rev/Fwd": Value Change {
        # "When the test mode helper value for relays is set, update that\ntree row item's value"
        n241 = event-data() -> ("NewVal.Forward"=w371:bool, "NewVal.Reverse"=w370:bool)  [unwired: 1 in]
        n242 = Boolean To (0,1)(Boolean=w371) -> (0, 1=w367:i16)
        n243 = Boolean To (0,1)(Boolean=w370) -> (0, 1=w369:i16)
        n244 = Negate(x=w369) -> (-x=w368:i16)
        n245 = Add(x=w367, y=w368) -> (x+y=w366:i16)
        n246 = call <vilib>:"NT Write Number.vi"("Numeric"=w366, "Name"=w365) -> ()  [unwired: 9 in, 1 out]
      }
      event "Test Ring": Value Change {
        # "When a test mode helper value is selected from the ring,\nset the tree item's variable to the string value"
        n247 = event-data() -> ("NewVal"=w375:u16)  [unwired: 1 in]
        n248 = property on="Test Ring" class="Ring (strict)"() -> ("Strings []"=w376:string[])  [unwired: 2 in, 2 out]
        n249 = Index Array(array=w376, index=w375) -> (element=w374:string)
        n250 = call <vilib>:"NT Write String.vi"("String"=w374, "Name"=w373) -> ()  [unwired: 9 in, 1 out]
      }
      event "Rec Mode": Value Change {
        # "Update globals for recording mode and path to read log from.\nClear when logging and let NetworkTables set path for vision to\nuse."
        n251 = event-data() -> ("NewVal"=w386:enum32{"Stop", "Record", "Playback"})  [unwired: 1 in]
        n252 = global write "WPI_DashboardLogging Global.vi" "Logging Filename"(path "") -> ()
        n253 = case shown="\"Playback\"" w386 {
          tunnel: w385 -> [_ w388 w396]
          tunnel: [_ _ w395] -> w382
          tunnel: [_ _ w394] -> _
          tunnel: w380 -> [_ _ w392]
          tunnel: cluster{i32, i32} {-250, 170} -> [_ _ w391]
          tunnel: [_ _ T23 {"Image Size"=TRUE, "Image Type"=TRUE, "Pixel Value"=TRUE, "ROI Information"=TRUE, "Zoom Factor"=FALSE} ("Image Information Shown:All Elements")] -> w378
          tunnel: [_ _ TRUE ("Zoom Factor")] -> w377
          frame Default {
          }
          frame "Stop", "Record" {
            # "Place Window too"
            n254 = invoke class="VI" method="FP.Close"(reference=w388) -> (reference out=w387:refnum<vi>)  [unwired: 2 in, 2 out]
            n255 = invoke class="VI" method="Abort VI"(reference=w387) -> ()  [unwired: 2 in, 3 out]
          }
          frame "Playback" {
            n256 = call "Open Playback Panel.vi"("Offset"=w391, "DB VI Ref"=w392, "Playback in"=w396) -> ("Playback out"=w393:refnum<vi>)  [unwired: 8 in]
            n257 = register-events(w393) -> (reference out=w395:refnum<event-registration>, error out=w394:errorcluster)  [unwired: 2 in]
          }
        }
        n258 = global write "WPI_DashboardLogging Global.vi" "Recording"(w386) -> ()
        n259 = property on="Camera Image" class="ImageControl"("Image Information Shown"=w378, "Image Information Visible"=w377) -> ()  [unwired: 2 in, 2 out]
        n260 = call <vilib>:"WPI_DashboardNT Log FieldName Cache.vi"("Operation"=enum16{"Lookup/Add", "Index", "Clear"}."Clear") -> ()  [unwired: 8 in, 3 out]
      }
      event Panel Close {
        w397 = enum32{"Stop", "Record", "Playback"}."Stop" ("Rec Mode")
        # "Playback window has been closed, abort"
        n261 = event-data() -> ()  [unwired: 1 in, 4 out]
        n262 = local write "Rec Mode"(w397) -> ()
        n263 = global write "WPI_DashboardLogging Global.vi" "Recording"(w397) -> ()
      }
      event Panel Close {
        # "Abort playback window and ourself"
        n264 = event-data() -> ()  [unwired: 1 in, 4 out]
        n265 = invoke class="VI" method="FP.Close"(reference=w402) -> (reference out=w401:refnum<vi>)  [unwired: 2 in, 2 out]
        n266 = invoke class="VI" method="Abort VI"(reference=w401) -> (error out=w400:errorcluster)  [unwired: 2 in, 2 out]
        n267 = invoke class="VI" method="Abort VI"(error in=w400) -> ()  [unwired: 2 in, 3 out]
      }
      event "Vision": Value Change {
        # "Enable/Disable Compression slider.\nHW USB is hard-coded into the camera"
        n268 = event-data() -> ("NewVal"=w408:u16)  [unwired: 1 in]
        n269 = Equal?(x=w408, y=u32 2 ("milliseconds to wait")) -> (x = y?=w406:bool)
        n270 = Select(t=T24."Disabled and Grayed Out" ("Disabled"), s=w406, f=T24."Enabled" ("Disabled")) -> (s? t:f=w403:T24)
        n271 = property on="Compression" class="Slide (strict)"("DisabledEnum"=w403) -> ()  [unwired: 2 in, 2 out]
      }
    }
  }
  n272 = while {
    tunnel: w23 -> [w411]
    i -> [w414]
    stop <- FALSE stop-if-true
    n273 = Wait (ms)(milliseconds to wait=u32 100) -> ()  [unwired: 1 out]
    n274 = case shown="\"Playback\"" "Rec Mode" {
      tunnel: w414 -> [_ _ w429]
      tunnel: [u32 2829099 ("Base Color") u32 11141120 ("Target Color") w418] -> w410
      frame "Stop", Default {
        # "Reset the color, extra updates don't cost much"
      }
      frame "Record" {
      }
      frame "Playback" {
        # "Playback"
        n275 = Quotient & Remainder(x=w429, y=u32 50 ("milliseconds to wait")) -> (x-y*floor(x/y)=w425:u32)  [unwired: 1 out]
        n276 = Divide(x=w425, y=u32 50 ("milliseconds to wait")) -> (x/y=w422:dbl)
        n277 = Multiply(x=6.283185307179586, y=w422) -> (x*y=w427:dbl)
        n278 = Sine(x=w427) -> (sin(x)=w426:dbl)
        n279 = Absolute Value(x=w426) -> (abs(x)=w419:dbl)
        n280 = call "Interpolate RGB Color.vi"("Proportion"=w419, "Target Color"=u32 30976, "Base Color"=u32 2829099) -> ("Result Color"=w418:u32)  [unwired: 8 in]
      }
    }
    n281 = property class="Pane"(reference=w411, "PaneColor"=w410) -> ()  [unwired: 1 in, 2 out]
  }
  n282 = TCP Create Listener(10:u16 1741 ("timeout ms (25000)")) -> (3:w1:refnum<k5>)  [unwired: 4 in, 2 out]
  n283 = while {
    tunnel: w1 -> [w431]
    stop <- FALSE stop-if-true
    n284 = TCP Wait On Listener(11:w431) -> (4:w430:refnum<k5>)  [unwired: 3 in, 4 out]
    n285 = local write "TCP"(w430) -> ()
  }
  n286 = property on="On/Off" class="Bool (strict)"("Visible"=w6) -> ()  [unwired: 2 in, 2 out]
  n287 = property on="Motor" class="Clust (strict)"("Visible"=w6) -> ()  [unwired: 2 in, 2 out]
  n288 = property on="Progress" class="Clust (strict)"("Visible"=w6) -> ()  [unwired: 2 in, 2 out]
  n289 = property on="Test Ring" class="Ring (strict)"("Visible"=w6) -> ()  [unwired: 2 in, 2 out]
  n290 = property on="Rev/Fwd" class="Clust (strict)"("Visible"=w6) -> ()  [unwired: 2 in, 2 out]
  n291 = property on="Camera Settings" class="Clust (strict)"("Visible"=w6) -> ()  [unwired: 2 in, 2 out]
  n292 = local write "DB Camera Config"(w6) -> ()
  n293 = global write "WPI_DashboardLogging Global.vi" "Recording"(w17) -> ()
  n294 = local write "Rec Mode"(w17) -> ()
